vi "niRFUtil TRC Waveform to Trace (real wfm).vi"(7 "Real Waveform":T2 {"y" min=0 max=127 format="%.2f"; "dx" format="%^.2e"; "x0" format="%^.2e"}) -> (8 "Measurement Trace":T1 format="%.2f")   [LabVIEW 2015, in "niRFUtil.lvlib"]
doc: "(c) Copyright 2006, National Instruments, Inc. This VI may not be duplicated, sold, or distributed without written consent from National Instruments."
uses:
  niRFUtil.lvlib
  Includes/niRFUtil INC Real Waveform.ctl
  Includes/niRFUtil INC Real Array.ctl
  Includes/niRFUtil INC Trace.ctl
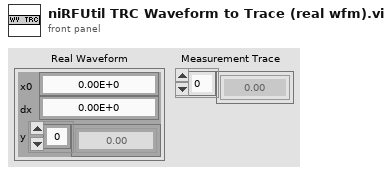
[diagram p1: front panel]
types:
  T1 = typedef "niRFUtil.lvlib/niRFUtil INC Trace.ctl" = sgl[]
  T2 = typedef "niRFUtil.lvlib/niRFUtil INC Real Waveform.ctl" = cluster{"x0":dbl, "dx":dbl, "y":T3}
  T3 = typedef "niRFUtil.lvlib/niRFUtil INC Real Array.ctl" = sgl[]
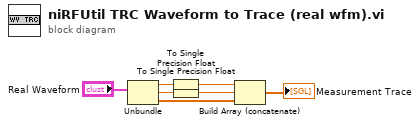
[diagram p0: block diagram]
diagram:
  n1 = Unbundle("Real Waveform") -> ("x0"=w7:dbl, "dx"=w6:dbl, "y"=w4:T3)
  n2 = To Single Precision Float(number=w7) -> (single precision float=w2:sgl)
  n3 = To Single Precision Float(number=w6) -> (single precision float=w1:sgl)
  n4 = Build Array (concatenate)(w2, w1, w4) -> (→"Measurement Trace":T3)
